vi "Grab with SW Trigger.vi"(10 "Trigger interval [ms]":u32, 11 "Camera Name\n(Test connection with NI MAX first)":refnum<k21> caption="IMAQdx Session") -> (0 "Error out":errorcluster caption="エラー出力", 2 "Time interval":i32(graph), 3 "Image (use SHIFT to unzoom)":T3(plugin-control))   [LabVIEW 2020]
doc: "The Low-Level Grab VI configures the number of buffers to use for the acquisition and configures an event callback to handle every other acquired image. A grab is appropriate for high-speed applications in which you need to process only one image at a time."
uses:
  <vilib>/vision/driver/IMAQdx.llb/IMAQdx Acquisition Mode.ctl
  Sub VIs and Controls/Timestamp FGV Command.ctl
  <vilib>/Utility/error.llb/DialogType.ctl
  <vilib>/vision/driver/IMAQdx.llb/IMAQdx Buffer Number Mode.ctl
  <vilib>/Analysis/baseanly.llb/Mean (DBL).vi
  <vilib>/Utility/error.llb/Error Cluster From Error Code.vi
  <vilib>/ErrorRing/Error Ring.xnode
  <resource>/objmgr/imaqdx.rc
  <vilib>/vision/driver/NI_Vision_Acquisition_Software.lvlib
  <vilib>/Analysis/NI_AALBase.lvlib
panel:
  in  "Save image to ...":path
  in  "Save image every ... seconds":i32
  in  "Set delimiter":string
  in  "Output mode":T1(ring)
  in  "Output file path":path
  in  "Log length (buffer #)":i32=100000
  out "XYグラフ":cluster{dbl[], dbl[]}[](graph)
  out "Connected at":string
  out "Histogram Graph":T2(graph) caption="Brightness Histogram"
  out "Acquired Frames per Second":dbl
  in  "Packet Size\n(Set to <=1500 unless \nJumbo Packet is enabled)":u32
  out "Timestamp of last frame":timestamp
  out "Start time":timestamp
  out "Acquisition loop iter":i32 format="%010.0f"
  out "Trigger driving loop iter":i32 format="%010.0f"
  out "Buffer Number":u32
  in  "Stop":bool
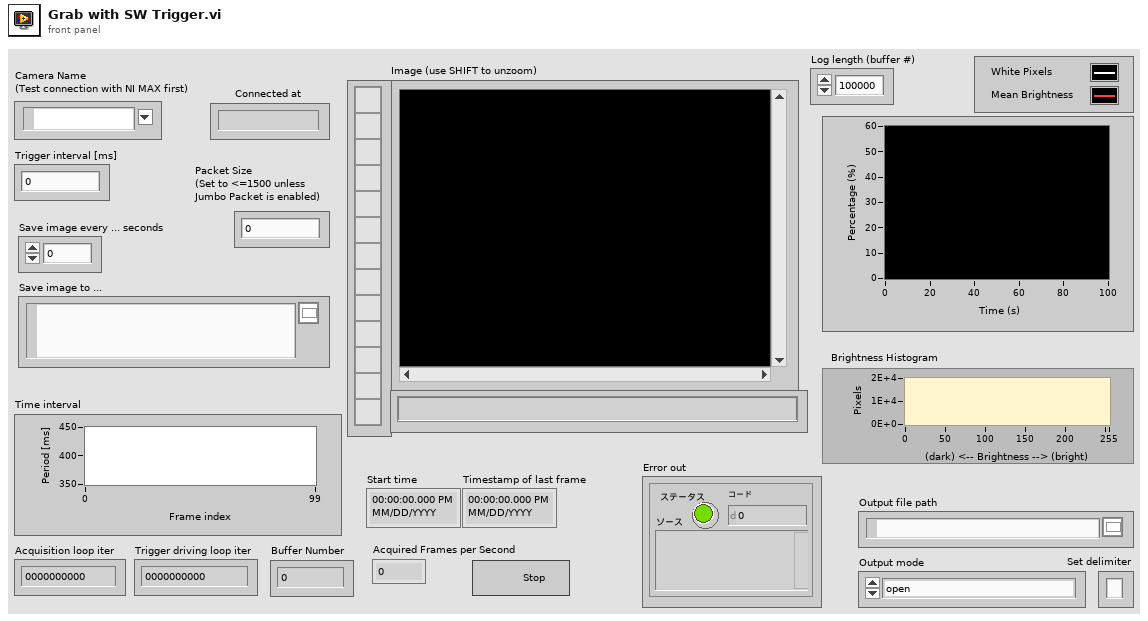
[diagram p1: front panel]
types:
  T1 = enum16{"open", "replace", "create", "open or create", "replace or create", "replace or create with confirmation"}
  T2 = cluster{"X Values":dbl[], "Histogram: h(x)":i32[]}
  T3 = typedef "IMAQ Image.ctl" = refnum<image>
  T4 = typedef "DialogType.ctl" = u16
  T5 = typedef "Timestamp FGV Command.ctl" = enum16{"Initialize", "Get"}
  T6 = typedef "NI_Vision_Acquisition_Software.lvlib/IMAQdx Acquisition Mode.ctl" = enum32{"One Shot", "Continuous"}
  T7 = typedef "IMAQdx.ctl" = refnum<k21>
  T8 = typedef "NI_Vision_Acquisition_Software.lvlib/IMAQdx Buffer Number Mode.ctl" = enum32{"Next", "Last", "Buffer Number", "Every", "Last New"}
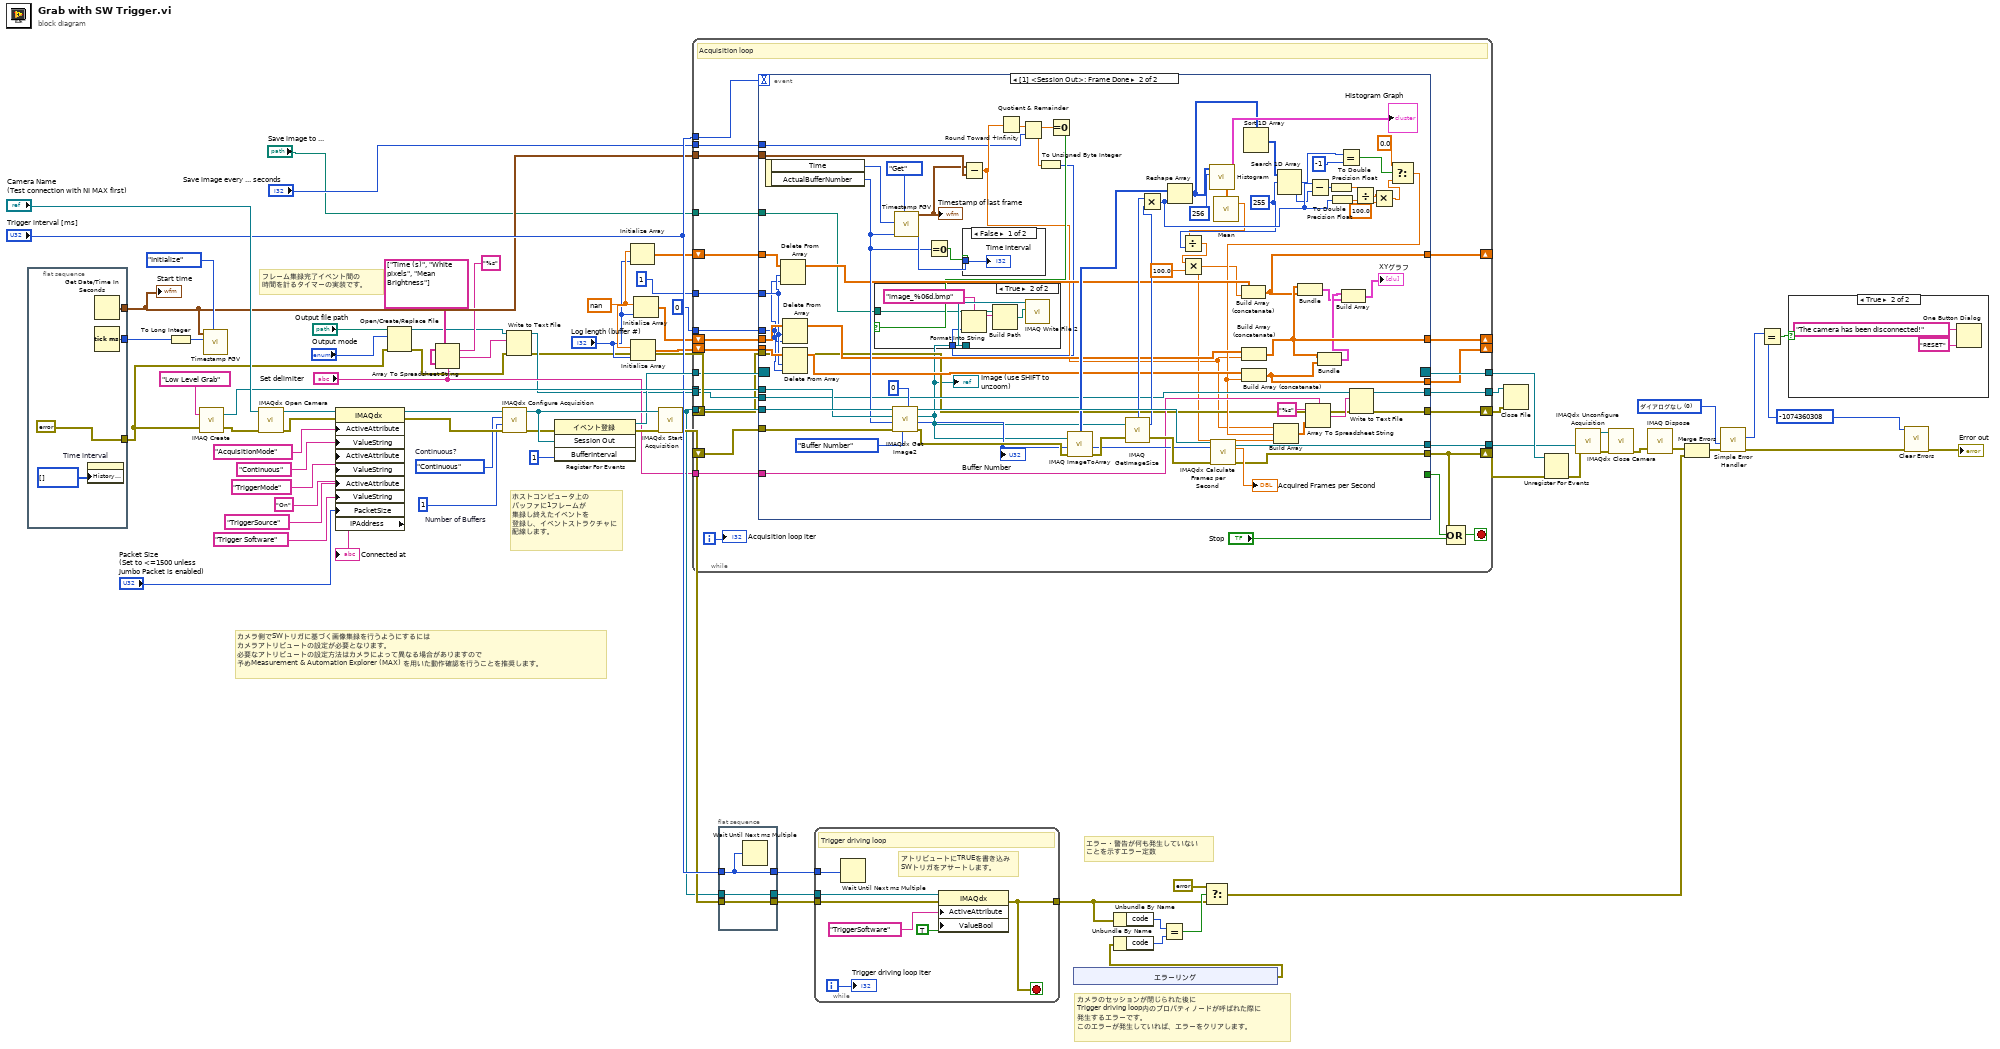
[diagram p0: block diagram]
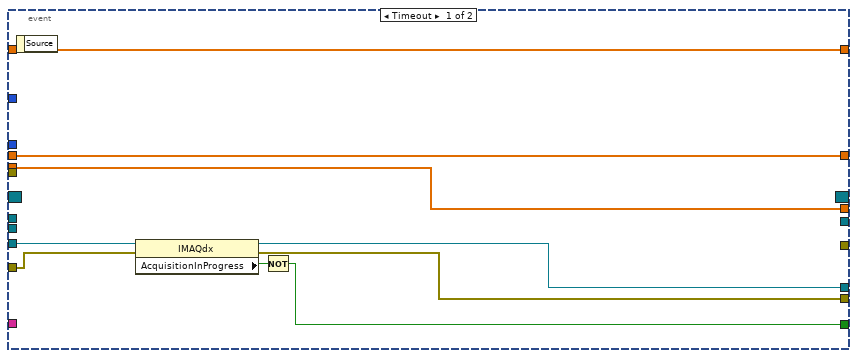
[diagram p3: hidden frame]
diagram:
  w10 = nan
  w28 = T4 0 items=["ダイアログなし", "OKメッセージ", "継続か停止メッセージ", "OKメッセージ+警告", "継続/停止+警告"] ("type of dialog (OK msg:1)")
  w25 = -1074360308
  w54 = u32 1  # Number of Buffers
  w53 = IMAQdx_Acquisition_Mode."Continuous"  # Continuous?
  # "エラー・警告が何も発生していない\nことを示すエラー定数"
  # "カメラのセッションが閉じられた後に\nTrigger driving loop内のプロパティノードが呼ばれた際に\n発生するエラーです。\nこのエラーが発生していれば、エラーをクリアします。"
  # "ホストコンピュータ上の\nバッファに1フレームが\n集録し終えたイベントを\n登録し、イベントストラクチャに\n配線します。"
  # "フレーム集録完了イベント間の\n時間を計るタイマーの実装です。"
  # "カメラ側でSWトリガに基づく画像集録を行うようにするには\nカメラアトリビュートの設定が必要となります。\n必要なアトリビュートの設定方法はカメラによって異なる場合がありますので\n予めMeasurement & Automation Explorer (MAX) を用いた動作確認を行うことを推奨します。"
  n1 = flat-sequence {
    tunnel: [w80] -> w39
    tunnel: [w79] -> w24
    tunnel: [errorcluster {"status"=FALSE, "code"=0, "source"=""} ("error in (no error)")] -> w3
    frame #0 {
      n2 = property on="Time interval" class="WFChart (指定)"("History Data"=i32[] [] ("履歴データ")) -> ()  [unwired: 2 in, 2 out]
      n3 = Get Date/Time In Seconds() -> (seconds since 1Jan1904=w79:timestamp)
      n4 = Tick Count (ms)() -> (millisecond timer value=w80:u32)
    }
  }
  n5 = To Long Integer(number=w39) -> (32bit integer=w40:i32)
  n6 = call "IMAQ Create"("Image Name"="Low Level Grab", "error in (no error)"=w3) -> ("New Image"=w50:T3, "error out"=w52:errorcluster)  [unwired: 2 in, 1 out]
  n7 = call "Timestamp FGV.vi"("Command"=Timestamp_FGV_Command."Initialize", "ms timer"=w40, "Previous frame timestamp"=w24) -> ()  [unwired: 7 in, 2 out]
  n8 = call <vilib>:"IMAQdx Open Camera.vi"("error in"=w52, "Session In"="Camera Name\n(Test connection with NI MAX first)") -> ("error out"=w62:errorcluster, "Session Out"=w61:T7)  [unwired: 1 in, 7 out]
  n9 = property class="IMAQdx"(reference=w61, error in=w62, "ActiveAttribute"="AcquisitionMode", "ValueString"="Continuous" ("ActiveAttribute"), "ActiveAttribute"="TriggerMode", "ValueString"="On" ("ActiveAttribute"), "ActiveAttribute"="TriggerSource", "ValueString"="Trigger Software" ("ActiveAttribute"), "PacketSize"="Packet Size\n(Set to <=1500 unless \nJumbo Packet is enabled)") -> (reference out=w64:T7, error out=w63:errorcluster, "IPAddress"=→"Connected at":string)
  n10 = Open/Create/Replace File(file path (use dialog)="Output file path", error in=w3, operation (0:open)="Output mode") -> (refnum out=w12:refnum<file>, error out=w7:errorcluster)  [unwired: 3 in, 1 out]
  n11 = Array To Spreadsheet String(delimiter (Tab)="Set delimiter", array=string[] ["Time (s)", "White pixels", "Mean Brightness"], 3:"%s" ("形式文字列")) -> (spreadsheet string=w16:string)
  n12 = call <vilib>:"IMAQdx Configure Acquisition.vi"("error in"=w63, "Number of Buffers"=w54, "Continuous?"=w53, "Session In"=w64) -> ("error out"=w55:errorcluster, "Session Out"=w57:T7)  [unwired: 6 out]
  n13 = Write to Text File(file (use dialog)=w12, text=w16, error in=w7) -> (refnum out=w11:refnum<file>, error out=w4:errorcluster)  [unwired: 1 in, 1 out]
  n14 = register-events(error in=w55, w57, u32 1 ("BufferInterval")) -> (reference out=w49:refnum<event-registration>, error out=w56:errorcluster)  [unwired: 1 in]
  n15 = Initialize Array(w10, "Log length (buffer #)") -> (w8:dbl[])
  n16 = Initialize Array(w10, "Log length (buffer #)") -> (w22:dbl[])
  n17 = Initialize Array(w10, "Log length (buffer #)") -> (w23:dbl[])
  n18 = call <vilib>:"IMAQdx Start Acquisition.vi"("error in"=w56, "Session In"=w57) -> ("error out"=w37:errorcluster, "Session Out"=w35:T7)  [unwired: 8 out]
  n19 = while {
    tunnel: "Trigger interval [ms]" -> [w105]
    tunnel: [w104] -> w76
    shift-right: [w106] -> w6
    shift-left: w37 -> [w108]
    tunnel: w35 -> [w103]
    tunnel: w50 -> [w102]
    tunnel: [w101] -> w45
    tunnel: w49 -> [w99]
    tunnel: w24 -> [w98]
    shift-right: [w95] -> _
    shift-left: w23 -> [w97]
    shift-right: [w93] -> _
    shift-left: w22 -> [w94]
    tunnel: 1 -> [w92]
    tunnel: 0 -> [w91]
    tunnel: "Set delimiter" -> [w88]
    shift-right: [w84] -> _
    shift-left: w8 -> [w87]
    tunnel: w11 -> [w90]
    tunnel: [w89] -> w17
    shift-right: [w86] -> w5
    shift-left: w4 -> [w85]
    tunnel: "Save image to ..." -> [w83]
    tunnel: "Save image every ... seconds" -> [w82]
    i -> [w96]
    stop <- w109 stop-if-true
    # "Acquisition loop"
    n20 = event shown="[1] <Session Out>: Frame Done" {
      selector: w99 -> [_ _]
      dyn-events: [_ _] -> w104
      timeout: w105 -> [_ _]
      tunnel: w108 -> [w116 w191]
      tunnel: [w115 w138] -> w106
      tunnel: w103 -> [w117 w190]
      tunnel: w102 -> [_ w189]
      tunnel: [w114 w183] -> w101
      tunnel: [w113 _] -> w100
      tunnel: w98 -> [_ w173]
      tunnel: w97 -> [w112 w171]
      tunnel: [w112 w155] -> w95
      tunnel: w94 -> [w111 w170]
      tunnel: [w111 w167] -> w93
      tunnel: w92 -> [_ w158]
      tunnel: w91 -> [_ w157]
      tunnel: w90 -> [_ w166]
      tunnel: [_ w165] -> w89
      tunnel: w88 -> [_ w163]
      tunnel: w87 -> [w110 w159]
      tunnel: [w110 w154] -> w84
      tunnel: [_ w137] -> w86
      tunnel: w85 -> [_ w136]
      tunnel: w83 -> [_ w122]
      tunnel: w82 -> [_ w119]
      event Timeout {
        n21 = event-data() -> ()  [unwired: 2 out]
        n22 = property class="IMAQdx"(reference=w117, error in=w116) -> (reference out=w114:T7, error out=w115:errorcluster, "AcquisitionInProgress"=w118:bool)
        n23 = Not(x=w118) -> (.not. x?=w113:bool)
      }
      event event #0x0 {
        w133 = u8 255 ("要素")
        n24 = event-data() -> ("Time"=w186:i32, "ActualBufferNumber"=w187:u32)  [unwired: 1 out]
        n25 = Delete From Array(array=w159, length=w158, index=w157) -> (array with subset deleted=w156:dbl[])  [unwired: 1 out]
        n26 = Delete From Array(array=w171, length=w158, index=w157) -> (array with subset deleted=w169:dbl[])  [unwired: 1 out]
        n27 = Delete From Array(array=w170, length=w158, index=w157) -> (array with subset deleted=w168:dbl[])  [unwired: 1 out]
        n28 = call <vilib>:"IMAQdx Get Image2.vi"("Timeout (ms)"=0, "Buffer Number Mode (Next)"=IMAQdx_Buffer_Number_Mode."Buffer Number" ("Buffer Number Mode"), "error in"=w191, "Buffer Number In"=w187, "Image In"=w189, "Session In"=w190) -> ("error out"=w179:errorcluster, "Buffer Number Out"=w172:u32, "Image Out"=w127:T3, "Session Out"=w184:T7)  [unwired: 2 in]
        "Image (use SHIFT to unzoom)" <- w127
        "Buffer Number" <- w172
        n29 = call "Timestamp FGV.vi"("Command"=Timestamp_FGV_Command."Get", "ActualBufferNumber"=w187, "ms timer"=w186) -> ("Time interval [ms]"=w194:i32, "Current frame timestamp"=w135:timestamp)  [unwired: 7 in]
        "Timestamp of last frame" <- w135
        n30 = Equal To 0?(x=w187) -> (x = 0?=w193:bool)
        n31 = Subtract(x=w135, y=w173) -> (x-y=w125:dbl)
        n32 = case "ケースストラクチャ" shown="FALSE" w193 {
          tunnel: w194 -> [w201 _]
          frame False {
            "Time interval" <- w201
          }
          frame True {
          }
        }
        n33 = Round Toward +Infinity(x=w125) -> (ceil(x): smallest int >= x=w124:dbl)
        n34 = Quotient & Remainder(x=w124, y=w119) -> (x-y*floor(x/y)=w123:dbl, floor(x/y)=w121:dbl)
        n35 = To Unsigned Byte Integer(number=w121) -> (unsigned 8bit integer=w120:u8)
        n36 = Equal To 0?(x=w123) -> (x = 0?=w126:bool)
        n37 = case shown="TRUE" w126 {
          tunnel: w127 -> [_ w200]
          tunnel: w122 -> [_ w197]
          tunnel: w120 -> [_ w195]
          frame False {
          }
          frame True {
            n38 = Format Into String(format string="image_%06d.bmp" ("形式文字列"), w195) -> (resulting string=w198:string)  [unwired: 2 in, 1 out]
            n39 = Build Path(base path=w197, name or relative path=w198) -> (appended path=w199:path)
            n40 = call-poly "IMAQ Write File 2"("File Path"=w199, "Image"=w200) -> ()  [unwired: 8 in, 2 out]
          }
        }
        n41 = call "IMAQ ImageToArray"("error in (no error)"=w179, "Image"=w127) -> ("error out"=w174:errorcluster, "Image Pixels (U8)"=w181:u8[][])  [unwired: 2 in, 3 out]
        n42 = call "IMAQ GetImageSize"("Image"=w127, "error in (no error)"=w174) -> ("Y Resolution"=w178:i32, "X Resolution"=w177:i32, "error out"=w176:errorcluster)  [unwired: 2 in]
        n43 = Multiply(x=w177, y=w178) -> (x*y=w146:i32)
        n44 = Reshape Array(w181, w146) -> (w160:u8[])
        n45 = call <vilib>:"Histogram.vi"("intervals"=256, "X"=w160) -> ("X Values"=w134:dbl[], "Histogram Graph"=→"Histogram Graph":T2)  [unwired: 6 in, 2 out]
        n46 = call <vilib>:"IMAQdx Calculate Frames per Second.vi"("Session In"=w184, "Buffer Number"=w172, "error in (no error)"=w176) -> ("Session Out"=w183:T7, "Acquired Frames per Second"=→"Acquired Frames per Second":dbl, "error out"=w138:errorcluster)  [unwired: 6 in, 4 out]
        n47 = call-poly <vilib>:"Mean.vi"("X"=w134) -> ("mean"=w132:dbl)  [unwired: 1 out]
        n48 = Divide(x=w132, y=w133) -> (x/y=w131:dbl)
        n49 = Multiply(x=w131, y=100.0) -> (x*y=w129:dbl)
        n50 = Build Array (concatenate)(w156, w129) -> (w154:dbl[])
        n51 = Build Array (concatenate)(w169, w125) -> (w155:dbl[])
        n52 = Sort 1D Array(array=w160) -> (sorted array=w140:u8[])
        n53 = Search 1D Array(1D array=w140, element=w133) -> (index of element=w139:i32)  [unwired: 1 in]
        n54 = Bundle(w155, w154) -> (w128:cluster{dbl[], dbl[]})  [unwired: 1 in]
        n55 = Subtract(x=w146, y=w139) -> (x-y=w147:i32)
        n56 = To Double Precision Float(number=w147) -> (double precision float=w149:dbl)
        n57 = To Double Precision Float(number=w146) -> (double precision float=w148:dbl)
        n58 = Equal?(x=w139, y=-1) -> (x = y?=w144:bool)
        n59 = Divide(x=w149, y=w148) -> (x/y=w151:dbl)
        n60 = Multiply(x=w151, y=100.0) -> (x*y=w142:dbl)
        n61 = Select(t=0.0, s=w144, f=w142) -> (s? t:f=w141:dbl)
        n62 = Build Array (concatenate)(w168, w141) -> (w167:dbl[])
        n63 = Build Array(w125, w141, w129) -> (w161:dbl[])
        n64 = Array To Spreadsheet String(delimiter (Tab)=w163, array=w161, 3:"%s" ("形式文字列")) -> (spreadsheet string=w164:string)
        n65 = Bundle(w155, w167) -> (w152:cluster{dbl[], dbl[]})  [unwired: 1 in]
        n66 = Build Array(w152, w128) -> (→"XYグラフ":cluster{dbl[], dbl[]}[])
        n67 = Write to Text File(file (use dialog)=w166, text=w164, error in=w136) -> (refnum out=w165:refnum<file>, error out=w137:errorcluster)  [unwired: 1 in, 1 out]
      }
    }
    n68 = Compound Arithmetic op=OR(w106, w100, "Stop") -> (w109:bool)
    "Acquisition loop iter" <- w96
  }
  n69 = flat-sequence {
    tunnel: [w204] -> w42
    tunnel: "Trigger interval [ms]" -> [w204]
    tunnel: w37 -> [w203]
    tunnel: [w203] -> w36
    tunnel: w35 -> [w202]
    tunnel: [w202] -> w34
    frame #0 {
      n70 = Wait Until Next ms Multiple(millisecond multiple=w204) -> ()  [unwired: 1 out]
    }
  }
  n71 = while {
    tunnel: [w206] -> w71
    tunnel: w34 -> [w208]
    tunnel: w36 -> [w205]
    tunnel: w42 -> [w207]
    i -> [w209]
    stop <- w206 stop-if-true
    # "アトリビュートにTRUEを書き込み\nSWトリガをアサートします。"
    # "Trigger driving loop"
    n72 = Wait Until Next ms Multiple(millisecond multiple=w207) -> ()  [unwired: 1 out]
    n73 = property class="IMAQdx"(reference=w208, error in=w205, "ActiveAttribute"="TriggerSoftware", "ValueBool"=TRUE) -> (error out=w206:errorcluster)  [unwired: 1 out]
    "Trigger driving loop iter" <- w209
  }
  n74 = xnode "エラーリング"() -> ("エラー出力"=w75:errorcluster)
  n75 = Unbundle By Name(w71) -> ("code"=w74:i32)
  n76 = Unbundle By Name(w75) -> ("code"=w73:i32)
  n77 = Equal?(x=w74, y=w73) -> (x = y?=w72:bool)
  n78 = Select(t=errorcluster {"status"=FALSE, "code"=0, "source"=""}, s=w72, f=w71) -> (s? t:f=w69:errorcluster)
  n79 = Close File(refnum=w17, error in=w5) -> ()  [unwired: 2 out]
  n80 = Unregister For Events(event registration refnum=w76, error in=w6) -> (error out=w46:errorcluster)
  n81 = call <vilib>:"IMAQdx Unconfigure Acquisition.vi"("error in"=w46, "Session In"=w45) -> ("error out"=w48:errorcluster, "Session Out"=w47:T7)  [unwired: 8 out]
  n82 = call <vilib>:"IMAQdx Close Camera.vi"("error in"=w48, "Session In"=w47) -> ("error out"=w44:errorcluster)  [unwired: 9 out]
  n83 = call "IMAQ Dispose"("error in (no error)"=w44) -> ("error out"=w43:errorcluster)  [unwired: 5 in]
  n84 = Merge Errors(w43, w69) -> (w31:errorcluster)
  n85 = call <vilib>:"Simple Error Handler.vi"("type of dialog (OK msg:1)"=w28, "error in (no error)"=w31) -> ("code out"=w30:i32, "error out"=w27:errorcluster)  [unwired: 3 in, 3 out]
  n86 = Equal?(x=w30, y=w25) -> (x = y?=w29:bool)
  n87 = case shown="TRUE" w29 {
    frame False {
    }
    frame True {
      n88 = One Button Dialog(message="The camera has been disconnected!" ("メッセージ"), button name ("OK")="RESET" ("ボタン名 (\"OK\")")) -> ()  [unwired: 1 out]
    }
  }
  n89 = call <vilib>:"Clear Errors.vi"("error in (no error)"=w27, "specific error code to clear (0: all)"=w25) -> ("error out"=→"Error out":errorcluster)  [unwired: 4 in, 1 out]
  "Start time" <- w24
